vi "Get Method List Column Ordering - Standard.vi"(8 "error in (no error)":errorcluster {"code" format="Error %.0f"}, 11 "VIDoc Printer - Confluence In":refnum<class "VIDoc Printer - Confluence.lvclass">) -> (0 "error out":errorcluster {"code" format="Error %.0f"}, 2 "Standard":T1[](array[typedef]), 3 "VIDoc Printer - Confluence Out":refnum<class "VIDoc Printer - Confluence.lvclass">)   [LabVIEW 2023, in "VIDoc Printer - Confluence.lvlib" / "VIDoc Printer - Confluence.lvclass"]
uses:
  VIDoc Printer - Confluence.lvclass
  Settings/Confluence Printer Settings/VI Info Column.ctl
  VIDoc Printer - Confluence.lvclass/VIDoc Printer - Confluence.ctl
  Settings/Confluence Printer Settings/VIDoc Settings - Confluence.lvclass
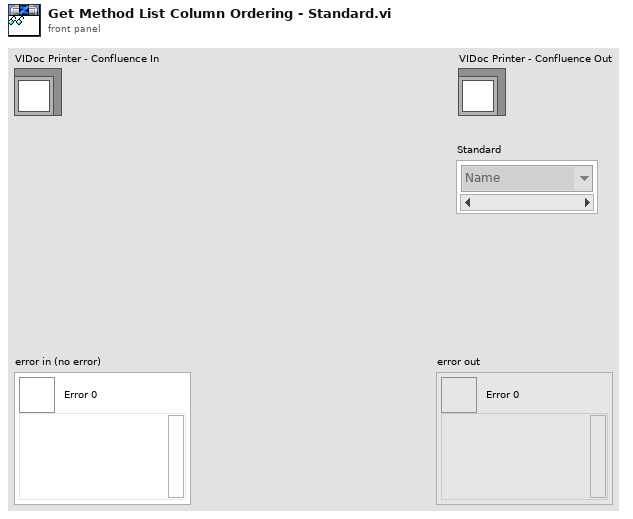
[diagram p1: front panel]
types:
  T1 = typedef "VIDoc Printer - Confluence.lvlib/VIDoc Settings - Confluence.lvclass/VI Info Column.ctl" = enum16{"Name", "Conpane", "BD", "FP", "VI Icon", "Description", "Reentrant", "Inline", "Auto Error", "Compiled", "Code Complexity", "Data Size", "Debug", "Priority", "Rev", "Minimum Size", "Title", "FP Behavior", "FP Closeable", "Author", "Commit Hash", "Last Change", "Branch", "Scope", "Type", "Dispatch", "Must Override", "Must Use Parent", "Structure Tree"}
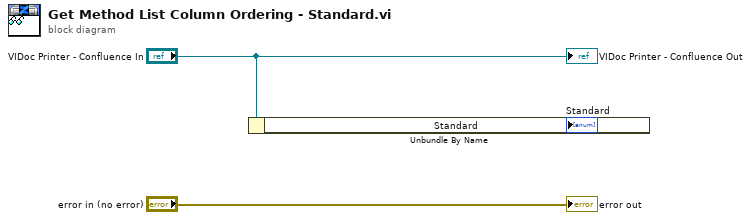
[diagram p0: block diagram]
diagram:
  n1 = Unbundle By Name("VIDoc Printer - Confluence In") -> ("Standard"=→"Standard":T1[])
  "error out" <- "error in (no error)"
  "VIDoc Printer - Confluence Out" <- "VIDoc Printer - Confluence In"
